vi "Pause.vi"(8 "error in (no error)":errorcluster, 11 "SS P100 Settings In":T1) -> (0 "error out":errorcluster, 3 "SS P100 Settings Out":T1)   [LabVIEW 2018, in "Sonic Systems P100.lvlib"]
uses:
  Sonic Systems P100.lvlib
  Sonic Systems P100 Settings.ctl
  support/Support Library.lvlib
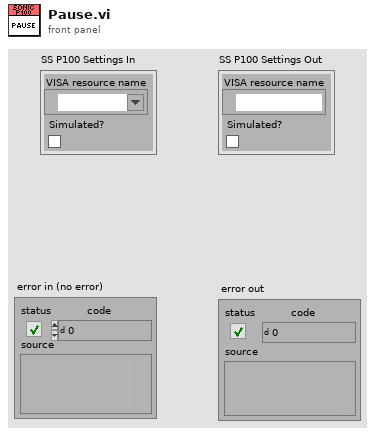
[diagram p1: front panel]
types:
  T1 = typedef "Sonic Systems P100.lvlib/Sonic Systems P100 Settings.ctl" = cluster{"VISA resource name":refnum<visa-resource-name>, "Simulated?":bool}
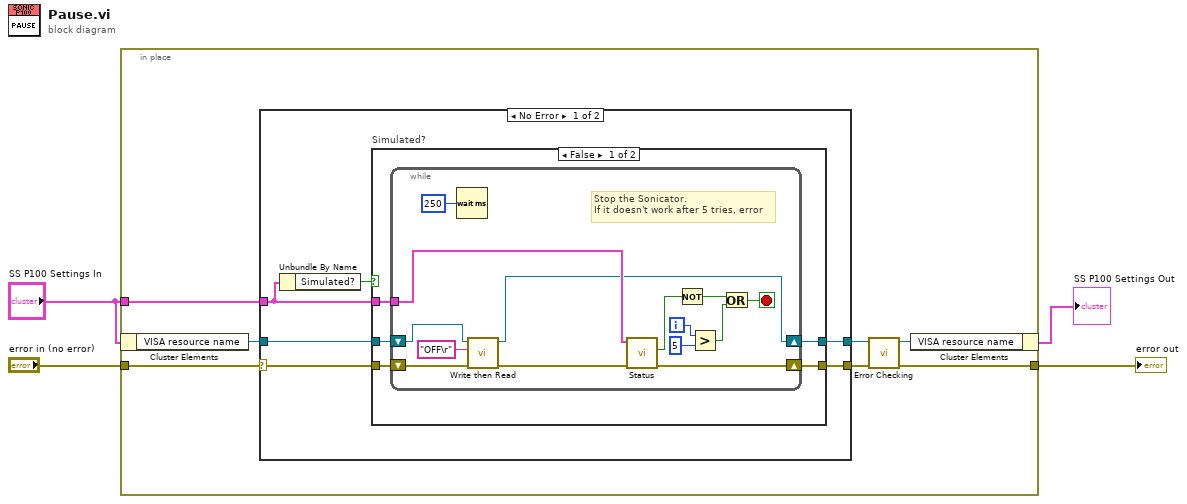
[diagram p0: block diagram]
diagram:
  n1 = in-place {
    in-place-border: "error in (no error)" -> [w11]
    in-place-border: [w8] -> w3
    in-place-border: "SS P100 Settings In" -> [w7]
    n2 = in-place-cluster #1("SS P100 Settings In") -> ("VISA resource name"=w6:refnum<visa-resource-name>)
    n3 = case shown="No Error" w11 {
      selector: w11 -> [w17 w40]
      tunnel: w7 -> [w13 _]
      tunnel: [w16 w40] -> w9
      tunnel: [w15 w39] -> w10
      tunnel: w6 -> [w12 w39]
      frame No Error {
        n4 = Unbundle By Name(w13) -> ("Simulated?"=w14:bool)
        n5 = case "Simulated?" shown="False" w14 {
          tunnel: w17 -> [w20 w38]
          tunnel: [w18 w38] -> w16
          tunnel: [w22 w37] -> w15
          tunnel: w12 -> [w21 w37]
          tunnel: w13 -> [w19 _]
          frame False {
            n6 = while {
              tunnel: w19 -> [w36]
              shift-right: [w25] -> w22
              shift-left: w21 -> [w29]
              shift-right: [w35] -> w18
              shift-left: w20 -> [w28]
              i -> [w33]
              stop <- w34 stop-if-true
              # "Stop the Sonicator. \nIf it doesn't work after 5 tries, error"
              n7 = Wait (ms)(milliseconds to wait=u32 250) -> ()  [unwired: 1 out]
              n8 = call "Write then Read.vi"("error in"=w28, "write buffer"="OFF\r" ("string"), "VISA resource name in"=w29) -> ("error out"=w26:errorcluster, "VISA resource name out"=w25:refnum<visa-resource-name>)  [unwired: 6 in, 1 out]
              n9 = call "Status.vi"("error in (no error)"=w26, "SS P100 Settings In"=w36) -> ("error out"=w35:errorcluster, "Running"=w23:bool)  [unwired: 4 in, 4 out]
              n10 = Not(x=w23) -> (.not. x?=w24:bool)
              n11 = Greater?(x=w33, y=5) -> (0:w31:bool)
              n12 = Or(x=w24, y=w31) -> (x .or. y?=w34:bool)
            }
          }
          frame True {
          }
        }
      }
      frame Error {
      }
    }
    n13 = call "Error Checking.vi"("error in (no error)"=w9, "VISA resource name"=w10) -> ("error out"=w8:errorcluster, "VISA resource name"=w5:refnum<visa-resource-name>)  [unwired: 7 in, 1 out]
    n14 = in-place-cluster #1("VISA resource name"=w5) -> (→"SS P100 Settings Out":T1)
  }
  "error out" <- w3
